vi "Get Response FIFO.vi"(11 "Interface in":refnum<class "Interface.lvclass">) -> (2 "Response FIFO":T1, 3 "Interface out":refnum<class "Interface.lvclass">)   [LabVIEW 2017, in "DSF Core.lvlib" / "Interface.lvclass"]
uses:
  Interface.lvclass
  RT FIFO Ref 16B.ctl
  RT FIFO Data 16B.ctl
  RT FIFO Payload 16B.ctl
  Interface.lvclass/Interface.ctl
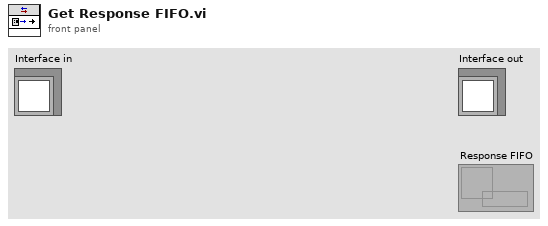
[diagram p1: front panel]
types:
  T1 = typedef "DSF Core.lvlib/Interface.lvclass/RT FIFO Ref 16B.ctl" = refnum<k33>
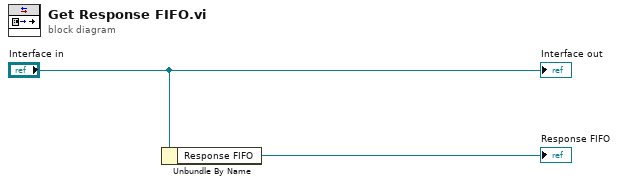
[diagram p0: block diagram]
diagram:
  n1 = Unbundle By Name("Interface in") -> ("Response FIFO"=→"Response FIFO":T1)
  "Interface out" <- "Interface in"
